vi "CopyOnly.vi"(8 "error in (no error)":errorcluster, 11 "ExistingFileMgr in":refnum<class "ExistingFileMgr.lvclass">) -> (0 "error out":errorcluster, 1 "EOF=T":bool, 2 "File Chunk to copy":string, 3 "ExistingFileMgr out":refnum<class "ExistingFileMgr.lvclass">, 5 "Next File Index":i64 format="%.9p", 7 "starting File Index":i64 format="%.9p")   [LabVIEW 2019, in "ExistingFileMgr.lvclass"]
doc: "When test execution is complete, if there is any data remaining in the pre-existing merge data file, then read it out to be copied it all over to the new file."
uses:
  ExistingFileMgr.lvclass
  ExistingFileMgr.lvclass/ExistingFileMgr.ctl
panel:
  out "size (bytes)":i64
  out "EndOfFile":bool
  out "error out 2":errorcluster
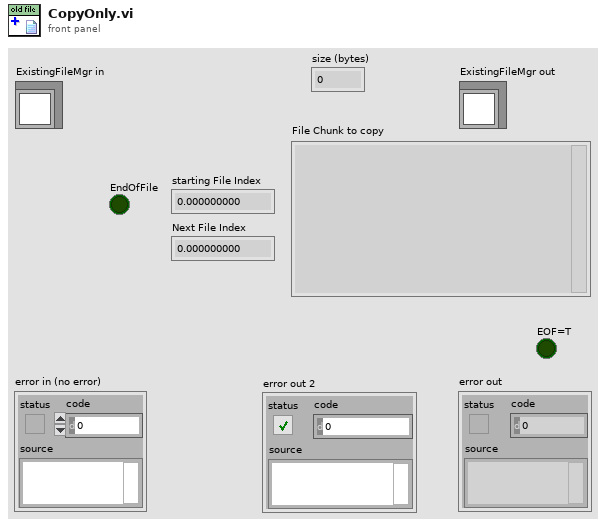
[diagram p1: front panel]
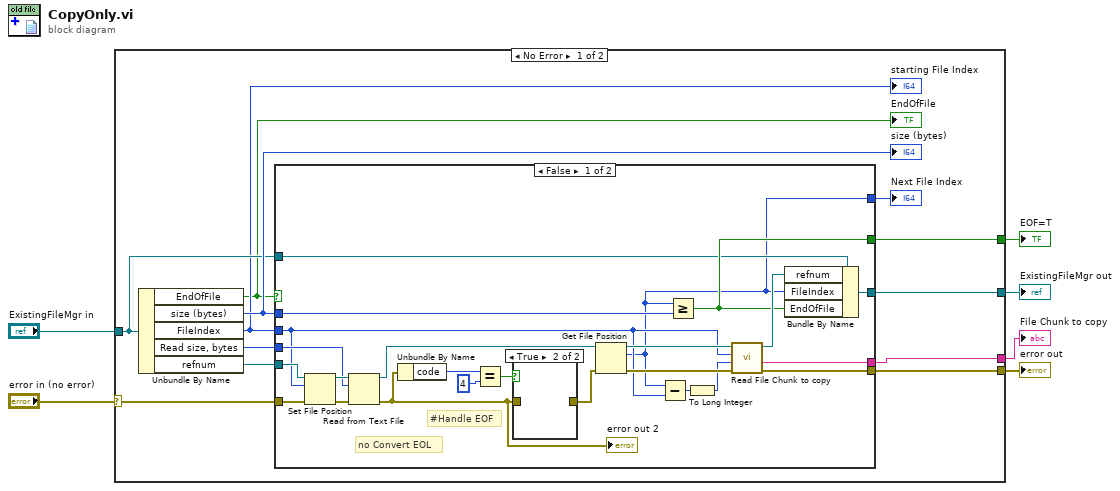
[diagram p0: block diagram]
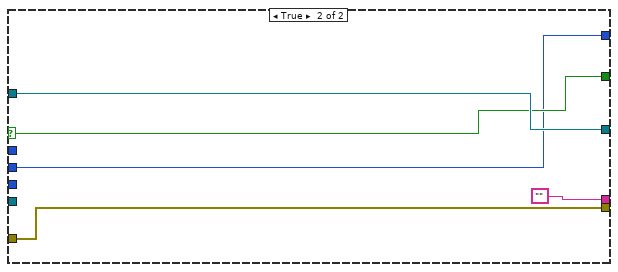
[diagram p3: hidden frame]
diagram:
  n1 = case shown="No Error" "error in (no error)" {
    selector: "error in (no error)" -> [w17 w50]
    tunnel: [w16 w50] -> w4
    tunnel: [w18 w49] -> w5
    tunnel: "ExistingFileMgr in" -> [w10 w49]
    tunnel: [w15 _] -> w2
    tunnel: [w11 _] -> w1
    frame No Error {
      n2 = Unbundle By Name(w10) -> ("EndOfFile"=w7:bool, "size (bytes)"=w14:i64, "FileIndex"=w9:i64, "Read size, bytes"=w12:i32, "refnum"=w13:refnum<file>)
      "starting File Index" <- w9
      "EndOfFile" <- w7
      "size (bytes)" <- w14
      n3 = case shown="False" w7 {
        selector: w7 -> [_ w47]
        tunnel: [w42 w48] -> w18
        tunnel: w17 -> [w37 w44]
        tunnel: [w35 w44] -> w16
        tunnel: [w34 ""] -> w15
        tunnel: w14 -> [w25 _]
        tunnel: w13 -> [w24 _]
        tunnel: w12 -> [w23 _]
        tunnel: [w22 w47] -> w11
        tunnel: w10 -> [w21 w48]
        tunnel: w9 -> [w20 w46]
        tunnel: [w19 w46] -> w8
        frame False {
          # "no Convert EOL"
          # "#Handle EOF"
          n4 = Set File Position(offset (in bytes) (0)=w20, refnum=w24, error in=w37) -> (refnum out=w39:refnum<file>, error out=w40:errorcluster)  [unwired: 1 in]
          n5 = Read from Text File(file (use dialog)=w39, count=w23, error in=w40) -> (refnum out=w38:refnum<file>, error out=w29:errorcluster)  [unwired: 1 in, 2 out]
          "error out 2" <- w29
          n6 = Unbundle By Name(w29) -> ("code"=w33:i32)
          n7 = Equal?(x=w33, y=4) -> (x = y?=w31:bool)
          n8 = case shown="True" w31 {
            tunnel: w29 -> [w43 _]
            tunnel: [w43 _] -> w30
            frame False {
            }
            frame True {
            }
          }
          n9 = Get File Position(4:w30, 7:w38) -> (0:w27:errorcluster, 2:w19:i64, 3:w36:refnum<file>)
          n10 = Subtract(x=w19, y=w20) -> (x-y=w28:i64)
          n11 = Greater Or Equal?(x=w19, y=w25) -> (x >= y?=w22:bool)
          n12 = To Long Integer(number=w28) -> (32bit integer=w26:i32)
          n13 = call "Read File Chunk to copy.vi"("error in"=w27, "Length to copy"=w26, "Start index"=w20, "refnum"=w36) -> ("error out"=w35:errorcluster, "File body to copy"=w34:string, "refnum out"=w41:refnum<file>)  [unwired: 5 in]
          n14 = Bundle By Name(cluster=w21, "refnum"=w41, "FileIndex"=w19, "EndOfFile"=w22) -> (w42:refnum<class "ExistingFileMgr.lvclass">)
        }
        frame True {
        }
      }
      "Next File Index" <- w8
    }
    frame Error {
    }
  }
  "error out" <- w4
  "ExistingFileMgr out" <- w5
  "File Chunk to copy" <- w2
  "EOF=T" <- w1
